vi "Set VI Object Save Setting.vi"(8 "error in (no error)":errorcluster, 10 "Remove compiled code":bool, 11 "NI_AB_API_Build in":refnum<class "NI_AB_API_Build.lvclass">) -> (0 "error out":errorcluster, 3 "NI_AB_API_Build out":refnum<class "NI_AB_API_Build.lvclass">)   [LabVIEW 2020, in "NI_AB_API_Build.lvclass"]
uses:
  <vilib>/AppBuilder/AB_API/Build/NI_AB_API_Build.lvclass
  <vilib>/AppBuilder/AB_API/Build/NI_AB_API_Build.lvclass/NI_AB_API_Build.ctl
  <vilib>/AppBuilder/AB_Classes/Build/AB_Build.lvclass
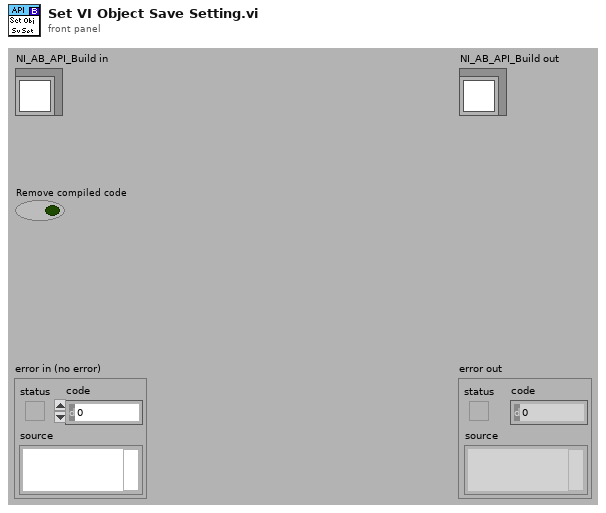
[diagram p1: front panel]
types:
  T1 = typedef "AB_Build.ctl" = cluster{"buildSpecName":string, "buildSpecDescription":string, "destinations":refnum<class "AB_Destination.lvclass">[], "exclusionOption":T2, "defaultLanguage":string, "supportedLanguages":string[], "excludedDirectories":path[], "buildContext":refnum<vi>, "buildObject":T3, "preview":bool, "programatic":bool, "progressBarEvents":T4, "userLog_Path":path, "preActionID":string, "preAction_Path":path, "postActionID":string, "postAction_Path":path, "eng_checkForBrokenVIs?":bool, "eng_verboseLinkerErrors?":bool, "localDest_Path":path, "targetDest_Path":path, "removeVIObject":u16, "cache":refnum<class "PreviewCache.lvclass">, "use cache":bool, "previewCache_ID":string, "buildCache_ID":string, "eng_TempLocalDest_Path":path, "eng_collectDependencies?":bool, "versionInfo":cluster{"buildVersion":cluster{"major":u16, "minor":u16, "patch":u16, "build":u16}, "autoIncrement":bool}, "eng_enableVIChecksums":bool}
  T2 = typedef "AB_Exclusion_Option.ctl" = cluster{"typedefs":bool, "polymorphicVIs":bool, "unusedLibraryItems":bool, "modifyLibraryFile":bool, "edit-timeDependencies":bool, "inlineVIs":bool, "dependent PPLs":bool, "dependent DLLs":bool}
  T3 = typedef "ItemRef.ctl" = u64
  T4 = typedef "provcom_ProgressBar_Events.ctl" = cluster{"newJob":refnum<user-event>, "newItem":refnum<user-event>, "errorMsg":T5, "cancel":refnum<user-event>}
  T5 = typedef "mxLvBuildError.ctl" = refnum<user-event>
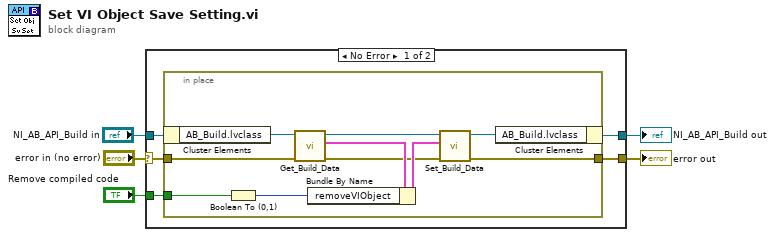
[diagram p0: block diagram]
diagram:
  n1 = case shown="No Error" "error in (no error)" {
    selector: "error in (no error)" -> [w9 w22]
    tunnel: [w10 w22] -> w4
    tunnel: [w6 w21] -> w2
    tunnel: "NI_AB_API_Build in" -> [w7 w21]
    tunnel: "Remove compiled code" -> [w8 _]
    frame No Error {
      n2 = in-place {
        in-place-border: [w20] -> w10
        in-place-border: w9 -> [w19]
        in-place-border: w8 -> [w18]
        n3 = in-place-cluster #1(w7) -> ("AB_Build.lvclass"=w12:refnum<class "AB_Build.lvclass">)
        n4 = Boolean To (0,1)(Boolean=w18) -> (0, 1=w11:i16)
        n5 = call <vilib>:"Get_Build_Data.vi"("error in (no error)"=w19, "Class in"=w12) -> ("error out"=w14:errorcluster, "data"=w16:T1, "Class out"=w17:refnum<class "AB_Build.lvclass">)  [unwired: 7 out]
        n6 = Bundle By Name(cluster=w16, "removeVIObject"=w11) -> (w15:T1)
        n7 = call <vilib>:"Set_Build_Data.vi"("error in (no error)"=w14, "data"=w15, "Class in"=w17) -> ("error out"=w20:errorcluster, "Class out"=w13:refnum<class "AB_Build.lvclass">)  [unwired: 7 out]
        n8 = in-place-cluster #1("AB_Build.lvclass"=w13) -> (w6:refnum<class "NI_AB_API_Build.lvclass">)
      }
    }
    frame Error {
    }
  }
  "error out" <- w4
  "NI_AB_API_Build out" <- w2
